vi "setup mfc usb interface.vi"(6 "co2 MFC max flow rate (mL/min)":dbl=500.0 format="%#_6p", 7 "Air MFC max flow rate (L/min)":dbl=5.0 format="%#_6p", 8 "error in":errorcluster, 9 "odor 2 MFC max flow rate (mL/min)":dbl=100.0 format="%#_6p", 10 "odor 1 MFC max flow rate (mL/min)":dbl=100.0 format="%#_6p", 11 "USB-6008 control channels":T2={"analog output channels"={"Dilution Air"="AirAndOdor1/ao0", "Odor 1"="AirAndOdor1/ao1", "Odor 2"="Odor2AndCO2/ao0", "CO2"="Odor2AndCO2/ao1"}, "analog input channels"={"air flow rate"="AirAndOdor1/ai0", "odor 1 flow rate"="AirAndOdor1/ai1", "odor 2 flow rate"="Odor2AndCO2/ai0", "co2 flow rate"="Odor2AndCO2/ai1", "pid sensor 1"="AirAndOdor1/ai2", "pid sensor 2"="AirAndOdor1/ai3"}, "digital control lines"={"air close"="AirAndOdor1/port0/line0", "air purge"="AirAndOdor1/port0/line1", "odor 1 close"="AirAndOdor1/port0/line2", "odor 1 purge"="AirAndOdor1/port0/line3", "odor 2 close"="Odor2AndCO2/port0/line0", "odor 2 purge"="Odor2AndCO2/port0/line1", "co2 close"="Odor2AndCO2/port0/line2", "co2 purge"="Odor2AndCO2/port0/line3"}}) -> (0 "error out":errorcluster, 3 "daqmx tasks":T1)   [LabVIEW 2013]
uses:
  <vilib>/DAQmx/write.llb/DAQmx Write (Digital Bool 1Line 1Point).vi
  <vilib>/DAQmx/create/scale.llb/DAQmx Create Scale (Linear).vi
  <vilib>/DAQmx/create/channels.llb/DAQmx Create Channel (AO-Voltage-Basic).vi
  <vilib>/DAQmx/create/channels.llb/DAQmx Create Channel (AI-Voltage-Basic).vi
  <vilib>/DAQmx/create/channels.llb/DAQmx Create Channel (DO-Digital Output).vi
  <vilib>/DAQmx/miscellaneous.llb/DAQmx Fill In Error Info.vi
panel:
  # "white = setpoint\nyellow = flow out\ngreen = valve off\nblue = purge"
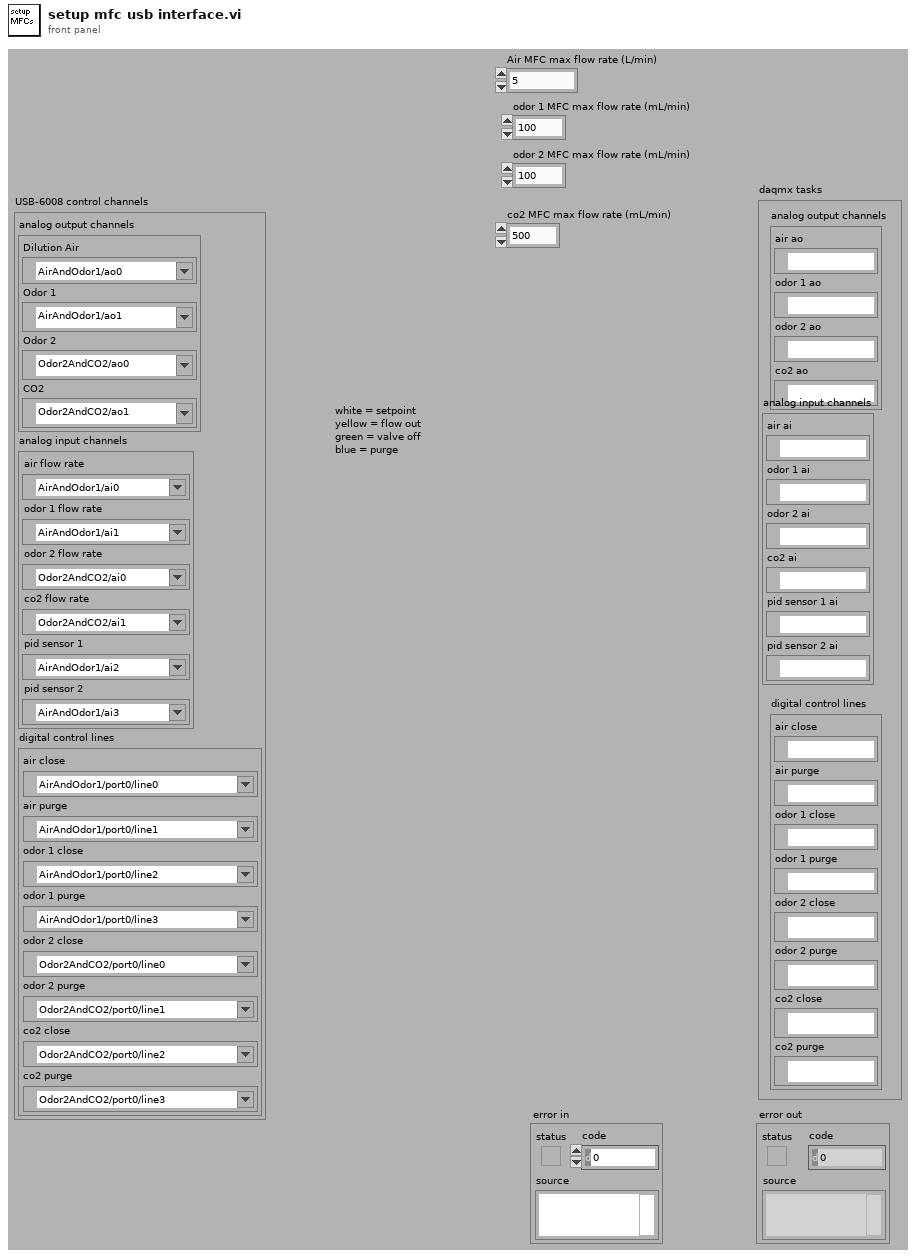
[diagram p1: front panel]
types:
  T1 = cluster{"analog output channels":cluster{"air ao":refnum<k21>, "odor 1 ao":refnum<k21>, "odor 2 ao":refnum<k21>, "co2 ao":refnum<k21>}, "analog input channels":cluster{"air ai":refnum<k21>, "odor 1 ai":refnum<k21>, "odor 2 ai":refnum<k21>, "co2 ai":refnum<k21>, "pid sensor 1 ai":refnum<k21>, "pid sensor 2 ai":refnum<k21>}, "digital control lines":cluster{"air close":refnum<k21>, "air purge":refnum<k21>, "odor 1 close":refnum<k21>, "odor 1 purge":refnum<k21>, "odor 2 close":refnum<k21>, "odor 2 purge":refnum<k21>, "co2 close":refnum<k21>, "co2 purge":refnum<k21>}}
  T2 = cluster{"analog output channels":cluster{"Dilution Air":tag, "Odor 1":tag, "Odor 2":tag, "CO2":tag}, "analog input channels":cluster{"air flow rate":tag, "odor 1 flow rate":tag, "odor 2 flow rate":tag, "co2 flow rate":tag, "pid sensor 1":tag, "pid sensor 2":tag}, "digital control lines":cluster{"air close":tag, "air purge":tag, "odor 1 close":tag, "odor 1 purge":tag, "odor 2 close":tag, "odor 2 purge":tag, "co2 close":tag, "co2 purge":tag}}
  T3 = cluster{"air close":refnum<k21>, "air purge":refnum<k21>, "odor 1 close":refnum<k21>, "odor 1 purge":refnum<k21>, "odor 2 close":refnum<k21>, "odor 2 purge":refnum<k21>, "co2 close":refnum<k21>, "co2 purge":refnum<k21>}
  T4 = cluster{"air ai":refnum<k21>, "odor 1 ai":refnum<k21>, "odor 2 ai":refnum<k21>, "co2 ai":refnum<k21>, "pid sensor 1 ai":refnum<k21>, "pid sensor 2 ai":refnum<k21>}
  T5 = cluster{"air ao":refnum<k21>, "odor 1 ao":refnum<k21>, "odor 2 ao":refnum<k21>, "co2 ao":refnum<k21>}
  T6 = cluster{"Dilution Air":tag, "Odor 1":tag, "Odor 2":tag, "CO2":tag}
  T7 = cluster{"air flow rate":tag, "odor 1 flow rate":tag, "odor 2 flow rate":tag, "co2 flow rate":tag, "pid sensor 1":tag, "pid sensor 2":tag}
  T8 = cluster{"air close":tag, "air purge":tag, "odor 1 close":tag, "odor 1 purge":tag, "odor 2 close":tag, "odor 2 purge":tag, "co2 close":tag, "co2 purge":tag}
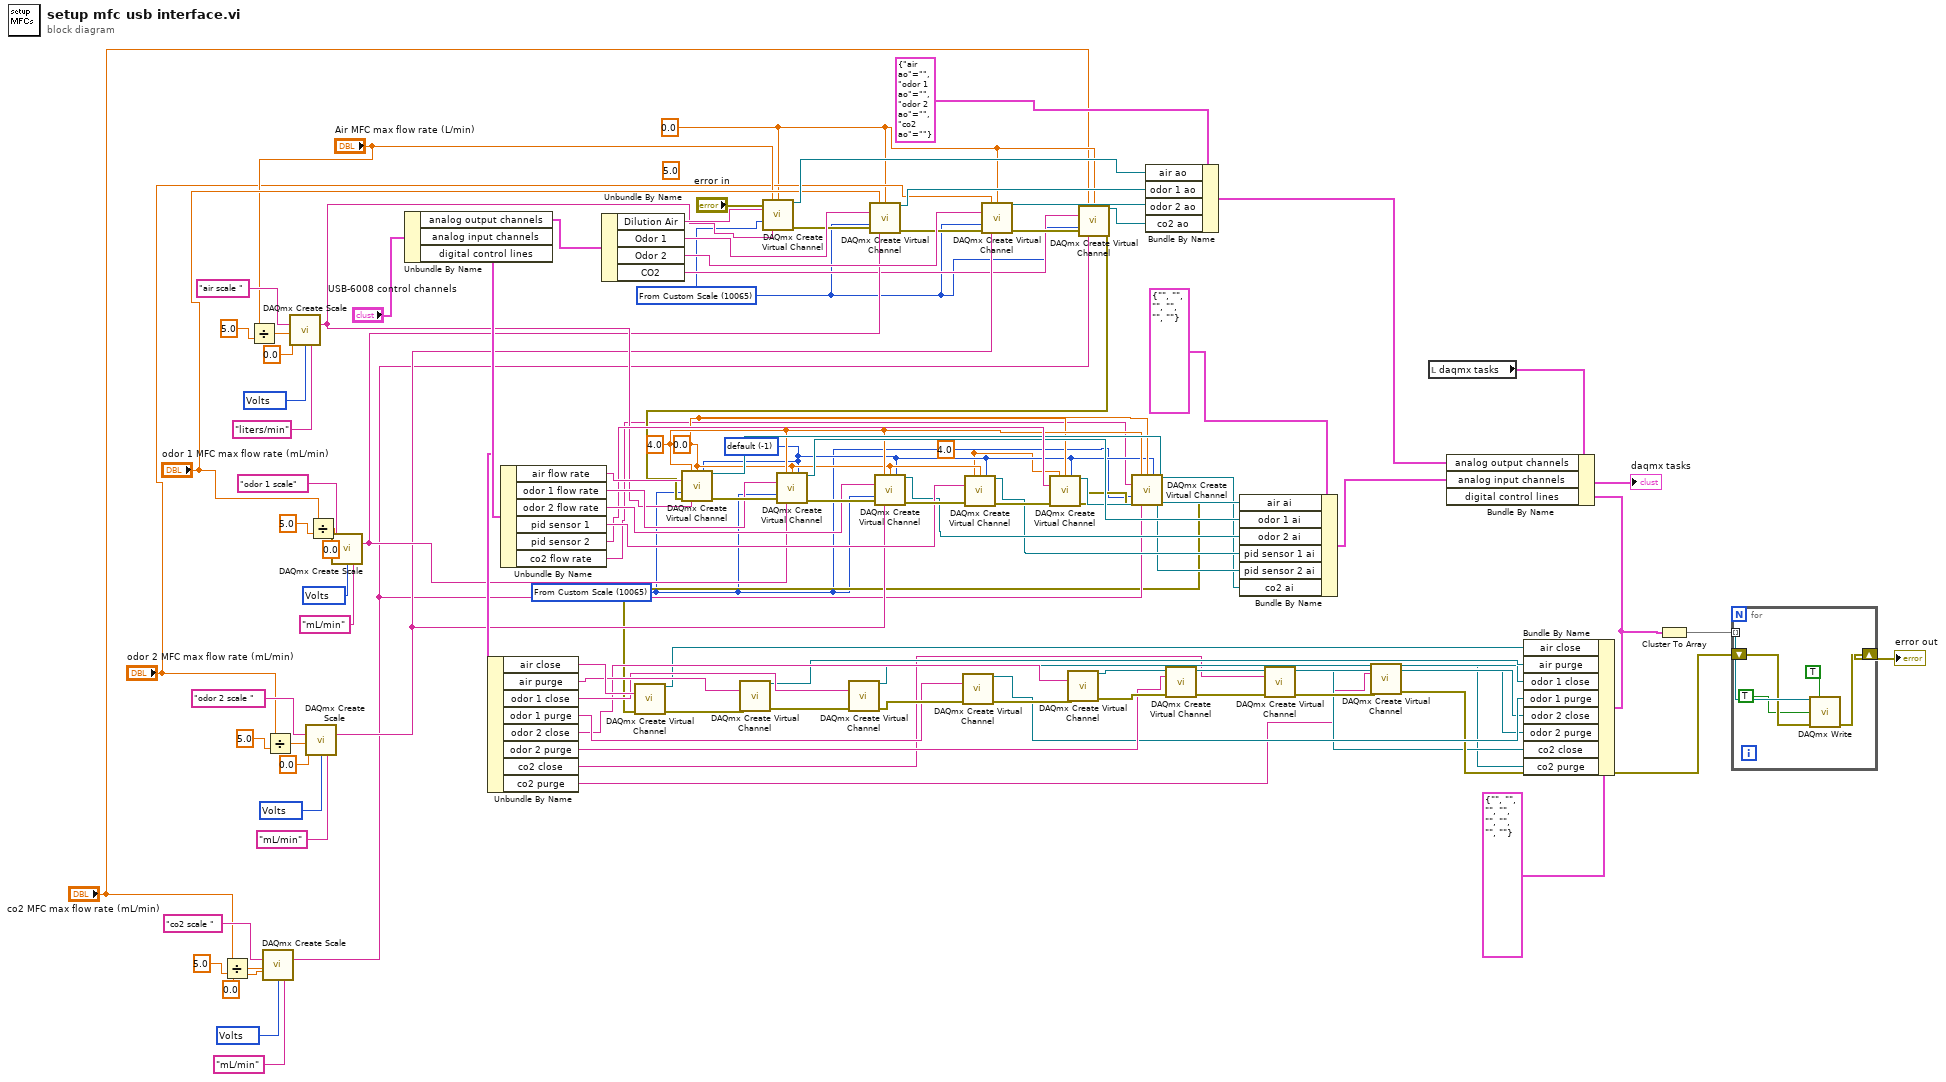
[diagram p0: block diagram]
diagram:
  w1 = 4.0 ("maximum value")
  w31 = 10348 items=["Volts"=10348, "Amps"=10342, "Deg F"=10144, "Deg C"=10143, "Deg R"=10145, "Kelvins"=10325, "Strain"=10299, "Ohms"=10384, "Hz"=10373, "Seconds"=10364, "Meters"=10219, "Inches"=10379, "Degrees"=10146, "Radians"=10273, "g"=10186, "m/s^2"=12470, "Pascals"=10081, "Newtons"=15875, "Pounds"=15876, "kgf"=15877, "psi"=15879, "bar"=15880, "Nm"=15881, "oz-in"=15882, "lb-in"=15883, "lb-ft"=15884, "Volts/Volt"=15896, "mVolts/Volt"=15897, "From TEDS"=12516] ("pre-scaled units")
  w16 = -1 items=["default"=-1, "RSE"=10083, "NRSE"=10078, "Differential"=10106, "Pseudodifferential"=12529] ("input terminal configuration")
  w2 = 10065 items=["Volts"=10348, "From Custom Scale"=10065] ("units")
  w44 = 10348 items=["Volts"=10348, "Amps"=10342, "Deg F"=10144, "Deg C"=10143, "Deg R"=10145, "Kelvins"=10325, "Strain"=10299, "Ohms"=10384, "Hz"=10373, "Seconds"=10364, "Meters"=10219, "Inches"=10379, "Degrees"=10146, "Radians"=10273, "g"=10186, "m/s^2"=12470, "Pascals"=10081, "Newtons"=15875, "Pounds"=15876, "kgf"=15877, "psi"=15879, "bar"=15880, "Nm"=15881, "oz-in"=15882, "lb-in"=15883, "lb-ft"=15884, "Volts/Volt"=15896, "mVolts/Volt"=15897, "From TEDS"=12516] ("pre-scaled units")
  w53 = 10348 items=["Volts"=10348, "Amps"=10342, "Deg F"=10144, "Deg C"=10143, "Deg R"=10145, "Kelvins"=10325, "Strain"=10299, "Ohms"=10384, "Hz"=10373, "Seconds"=10364, "Meters"=10219, "Inches"=10379, "Degrees"=10146, "Radians"=10273, "g"=10186, "m/s^2"=12470, "Pascals"=10081, "Newtons"=15875, "Pounds"=15876, "kgf"=15877, "psi"=15879, "bar"=15880, "Nm"=15881, "oz-in"=15882, "lb-in"=15883, "lb-ft"=15884, "Volts/Volt"=15896, "mVolts/Volt"=15897, "From TEDS"=12516] ("pre-scaled units")
  w3 = 10065 items=["Volts"=10348, "From Custom Scale"=10065] ("units")
  w60 = 10348 items=["Volts"=10348, "Amps"=10342, "Deg F"=10144, "Deg C"=10143, "Deg R"=10145, "Kelvins"=10325, "Strain"=10299, "Ohms"=10384, "Hz"=10373, "Seconds"=10364, "Meters"=10219, "Inches"=10379, "Degrees"=10146, "Radians"=10273, "g"=10186, "m/s^2"=12470, "Pascals"=10081, "Newtons"=15875, "Pounds"=15876, "kgf"=15877, "psi"=15879, "bar"=15880, "Nm"=15881, "oz-in"=15882, "lb-in"=15883, "lb-ft"=15884, "Volts/Volt"=15896, "mVolts/Volt"=15897, "From TEDS"=12516] ("pre-scaled units")
  w18 = 4.0 ("maximum value")
  w17 = 0.0 ("minimum value")
  (unwired) 5.0 ("Maximum Value")
  w21 = 0.0 ("Minimum Value")
  n1 = Divide(x="co2 MFC max flow rate (mL/min)", y=5.0 ("x")) -> (x/y=w34:dbl)
  n2 = Divide(x="Air MFC max flow rate (L/min)", y=5.0 ("x")) -> (x/y=w63:dbl)
  n3 = call-poly <vilib>:"DAQmx Create Scale.vi"("name"="co2 scale " ("air scale (L/min)"), "slope"=w34, "y-intercept"=0.0, "pre-scaled units"=w31, "scaled units"="mL/min") -> ("scale out"=w15:tag)  [unwired: 9 in, 1 out]
  n4 = Divide(x="odor 2 MFC max flow rate (mL/min)", y=5.0 ("x")) -> (x/y=w47:dbl)
  n5 = call-poly <vilib>:"DAQmx Create Scale.vi"("name"="air scale " ("air scale (L/min)"), "slope"=w63, "y-intercept"=0.0, "pre-scaled units"=w60, "scaled units"="liters/min") -> ("scale out"=w58:tag)  [unwired: 9 in, 1 out]
  n6 = call-poly <vilib>:"DAQmx Create Scale.vi"("name"="odor 2 scale " ("air scale (L/min)"), "slope"=w47, "y-intercept"=0.0, "pre-scaled units"=w44, "scaled units"="mL/min") -> ("scale out"=w41:tag)  [unwired: 9 in, 1 out]
  n7 = Divide(x="odor 1 MFC max flow rate (mL/min)", y=5.0 ("x")) -> (x/y=w56:dbl)
  n8 = call-poly <vilib>:"DAQmx Create Scale.vi"("name"="odor 1 scale" ("air scale (L/min)"), "slope"=w56, "y-intercept"=0.0, "pre-scaled units"=w53, "scaled units"="mL/min") -> ("scale out"=w42:tag)  [unwired: 9 in, 1 out]
  n9 = Unbundle By Name("USB-6008 control channels") -> ("analog output channels"=w103:T6, "analog input channels"=w89:T7, "digital control lines"=w78:T8)
  n10 = Unbundle By Name(w78) -> ("air close"=w77:tag, "air purge"=w76:tag, "odor 1 close"=w75:tag, "odor 1 purge"=w74:tag, "odor 2 close"=w73:tag, "odor 2 purge"=w72:tag, "co2 close"=w7:tag, "co2 purge"=w4:tag)
  n11 = Unbundle By Name(w89) -> ("air flow rate"=w88:tag, "odor 1 flow rate"=w87:tag, "odor 2 flow rate"=w86:tag, "pid sensor 1"=w85:tag, "pid sensor 2"=w84:tag, "co2 flow rate"=w14:tag)
  n12 = Unbundle By Name(w103) -> ("Dilution Air"=w102:tag, "Odor 1"=w101:tag, "Odor 2"=w100:tag, "CO2"=w23:tag)
  n13 = call-poly <vilib>:"DAQmx Create Virtual Channel.vi"("maximum value"="Air MFC max flow rate (L/min)", "minimum value"=w21, "physical channels"=w102, "units"=w3, "error in"="error in", "custom scale name"=w58) -> ("task out"=w99:refnum<k21>, "error out"=w92:errorcluster)  [unwired: 8 in]
  n14 = call-poly <vilib>:"DAQmx Create Virtual Channel.vi"("maximum value"="odor 1 MFC max flow rate (mL/min)", "minimum value"=w21, "physical channels"=w101, "units"=w3, "error in"=w92, "custom scale name"=w42) -> ("task out"=w98:refnum<k21>, "error out"=w91:errorcluster)  [unwired: 8 in]
  n15 = call-poly <vilib>:"DAQmx Create Virtual Channel.vi"("maximum value"="odor 2 MFC max flow rate (mL/min)", "minimum value"=w21, "physical channels"=w100, "units"=w3, "error in"=w91, "custom scale name"=w41) -> ("task out"=w97:refnum<k21>, "error out"=w25:errorcluster)  [unwired: 8 in]
  n16 = call-poly <vilib>:"DAQmx Create Virtual Channel.vi"("maximum value"="co2 MFC max flow rate (mL/min)", "minimum value"=w21, "physical channels"=w23, "units"=w3, "error in"=w25, "custom scale name"=w15) -> ("task out"=w19:refnum<k21>, "error out"=w24:errorcluster)  [unwired: 8 in]
  n17 = call-poly <vilib>:"DAQmx Create Virtual Channel.vi"("maximum value"=w18, "minimum value"=w17, "input terminal configuration"=w16, "physical channels"=w88, "units"=w2, "error in"=w24, "custom scale name"=w58) -> ("task out"=w83:refnum<k21>, "error out"=w96:errorcluster)  [unwired: 7 in]
  n18 = call-poly <vilib>:"DAQmx Create Virtual Channel.vi"("maximum value"=w18, "minimum value"=w17, "input terminal configuration"=w16, "physical channels"=w87, "units"=w2, "error in"=w96, "custom scale name"=w42) -> ("task out"=w82:refnum<k21>, "error out"=w95:errorcluster)  [unwired: 7 in]
  n19 = call-poly <vilib>:"DAQmx Create Virtual Channel.vi"("maximum value"=w18, "minimum value"=w17, "input terminal configuration"=w16, "physical channels"=w86, "units"=w2, "error in"=w95, "custom scale name"=w41) -> ("task out"=w81:refnum<k21>, "error out"=w94:errorcluster)  [unwired: 7 in]
  n20 = call-poly <vilib>:"DAQmx Create Virtual Channel.vi"("maximum value"=w1, "minimum value"=w17, "input terminal configuration"=w16, "physical channels"=w85, "error in"=w94) -> ("task out"=w80:refnum<k21>, "error out"=w93:errorcluster)  [unwired: 9 in]
  n21 = call-poly <vilib>:"DAQmx Create Virtual Channel.vi"("maximum value"=w1, "minimum value"=w17, "input terminal configuration"=w16, "physical channels"=w84, "error in"=w93) -> ("task out"=w79:refnum<k21>, "error out"=w12:errorcluster)  [unwired: 9 in]
  n22 = call-poly <vilib>:"DAQmx Create Virtual Channel.vi"("maximum value"=w18, "minimum value"=w17, "input terminal configuration"=w16, "physical channels"=w14, "units"=w2, "error in"=w12, "custom scale name"=w15) -> ("task out"=w13:refnum<k21>, "error out"=w11:errorcluster)  [unwired: 7 in]
  n23 = call-poly <vilib>:"DAQmx Create Virtual Channel.vi"("lines"=w77, "error in"=w11) -> ("task out"=w71:refnum<k21>, "error out"=w108:errorcluster)  [unwired: 12 in]
  n24 = call-poly <vilib>:"DAQmx Create Virtual Channel.vi"("lines"=w76, "error in"=w108) -> ("task out"=w70:refnum<k21>, "error out"=w107:errorcluster)  [unwired: 12 in]
  n25 = call-poly <vilib>:"DAQmx Create Virtual Channel.vi"("lines"=w75, "error in"=w107) -> ("task out"=w69:refnum<k21>, "error out"=w104:errorcluster)  [unwired: 12 in]
  n26 = call-poly <vilib>:"DAQmx Create Virtual Channel.vi"("lines"=w74, "error in"=w104) -> ("task out"=w68:refnum<k21>, "error out"=w106:errorcluster)  [unwired: 12 in]
  n27 = call-poly <vilib>:"DAQmx Create Virtual Channel.vi"("lines"=w73, "error in"=w106) -> ("task out"=w67:refnum<k21>, "error out"=w105:errorcluster)  [unwired: 12 in]
  n28 = Bundle By Name(cluster=T5 {"air ao"="", "odor 1 ao"="", "odor 2 ao"="", "co2 ao"=""} ("analog output channels"), "air ao"=w99, "odor 1 ao"=w98, "odor 2 ao"=w97, "co2 ao"=w19) -> (w50:T5)
  n29 = call-poly <vilib>:"DAQmx Create Virtual Channel.vi"("lines"=w72, "error in"=w105) -> ("task out"=w66:refnum<k21>, "error out"=w10:errorcluster)  [unwired: 12 in]
  n30 = Bundle By Name(cluster=T4 {"air ai"="", "odor 1 ai"="", "odor 2 ai"="", "co2 ai"="", "pid sensor 1 ai"="", "pid sensor 2 ai"=""} ("analog input channels"), "air ai"=w83, "odor 1 ai"=w82, "odor 2 ai"=w81, "pid sensor 1 ai"=w80, "pid sensor 2 ai"=w79, "co2 ai"=w13) -> (w49:T4)
  n31 = call-poly <vilib>:"DAQmx Create Virtual Channel.vi"("lines"=w7, "error in"=w10) -> ("task out"=w6:refnum<k21>, "error out"=w9:errorcluster)  [unwired: 12 in]
  n32 = call-poly <vilib>:"DAQmx Create Virtual Channel.vi"("lines"=w4, "error in"=w9) -> ("task out"=w5:refnum<k21>, "error out"=w8:errorcluster)  [unwired: 12 in]
  n33 = local read "daqmx tasks"() -> (w29:T1)
  n34 = Bundle By Name(cluster=T3 {"air close"="", "air purge"="", "odor 1 close"="", "odor 1 purge"="", "odor 2 close"="", "odor 2 purge"="", "co2 close"="", "co2 purge"=""} ("digital control lines"), "air close"=w71, "air purge"=w70, "odor 1 close"=w69, "odor 1 purge"=w68, "odor 2 close"=w67, "odor 2 purge"=w66, "co2 close"=w6, "co2 purge"=w5) -> (w38:T3)
  n35 = Bundle By Name(cluster=w29, "analog output channels"=w50, "analog input channels"=w49, "digital control lines"=w38) -> (→"daqmx tasks":T1)
  n36 = Cluster To Array(cluster=w38) -> (array=w37:refnum<k21>[])
  n37 = for {
    tunnel: w37 -> [w113] mode=indexing
    shift-right: [w111] -> w36
    shift-left: w8 -> [w112]
    n38 = call-poly <vilib>:"DAQmx Write.vi"("task/channels in"=w113, "auto start"=TRUE, "data"=TRUE ("auto start"), "error in"=w112) -> ("error out"=w111:errorcluster)  [unwired: 9 in, 2 out]
  }
  "error out" <- w36
